vi "Output on.vi"(8 "error in (no error)":errorcluster, 10 "Output On":bool, 11 "E364x in":refnum<class "E364x.lvclass">) -> (0 "error out":errorcluster, 3 "E364x out":refnum<class "E364x.lvclass">)   [LabVIEW 2020, in "E364x.lvclass"]
uses:
  E364x.lvclass
  C:/Sandbox/RF Bench/Source Code/WiSpry Test Framework/Instruments/Instrument.lvclass
  Instrument.lvclass/Instrument.ctl
  Instrument.lvclass
  <instrlib>/Agilent E364X Series/Agilent E364X Series.lvlib
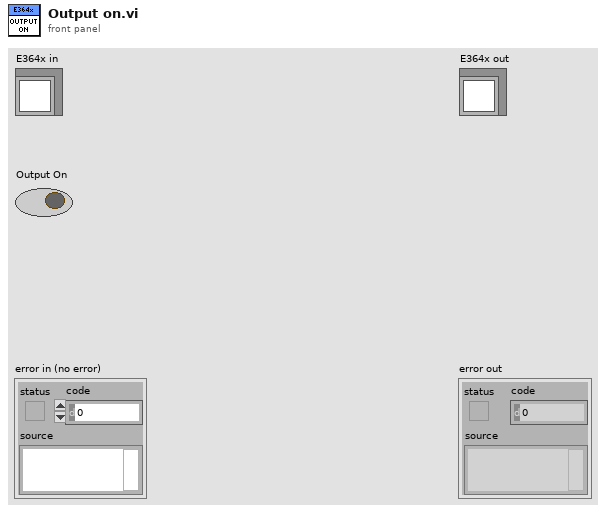
[diagram p1: front panel]
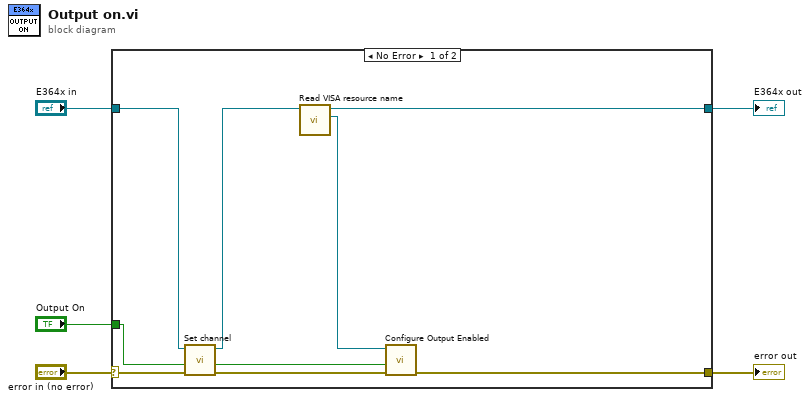
[diagram p0: block diagram]
diagram:
  n1 = case shown="No Error" "error in (no error)" {
    selector: "error in (no error)" -> [w9 w15]
    tunnel: [w12 w15] -> w1
    tunnel: [w10 w14] -> w2
    tunnel: "E364x in" -> [w7 w14]
    tunnel: "Output On" -> [w11 _]
    frame No Error {
      n2 = call "Set channel.vi"("error in (no error)"=w9, "E364x in"=w7) -> ("error out"=w8:errorcluster, "E364x out"=w6:refnum<class "E364x.lvclass">)  [unwired: 7 in, 1 out]
      n3 = call "Read VISA resource name.vi"("Instrument in"=w6) -> ("VISA resource name"=w13:refnum<visa-resource-name>, "Instrument out"=w10:refnum<class "E364x.lvclass">)  [unwired: 9 in]
      n4 = call <instrlib>:"Configure Output Enabled.vi"("error in (no error)"=w8, "Output Enabled (F: Off)"=w11, "VISA resource name"=w13) -> ("error out"=w12:errorcluster)  [unwired: 7 in, 1 out]
    }
    frame Error {
    }
  }
  "error out" <- w1
  "E364x out" <- w2
